vi "Convert Array_String to String.vi"(10 "Data 2":string[][](array[string]), 11 "Data 1":string[](array[string])) -> (3 "String Out":string)   [LabVIEW 2020, in "GUCalibration2.lvlib"]
uses:
  GUCalibration2.lvlib
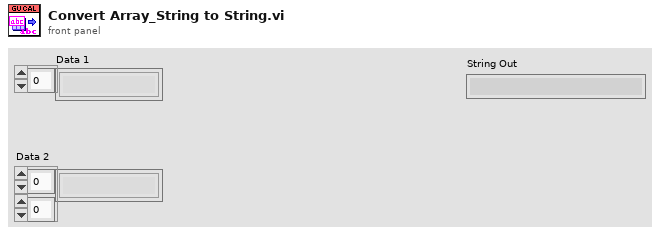
[diagram p1: front panel]
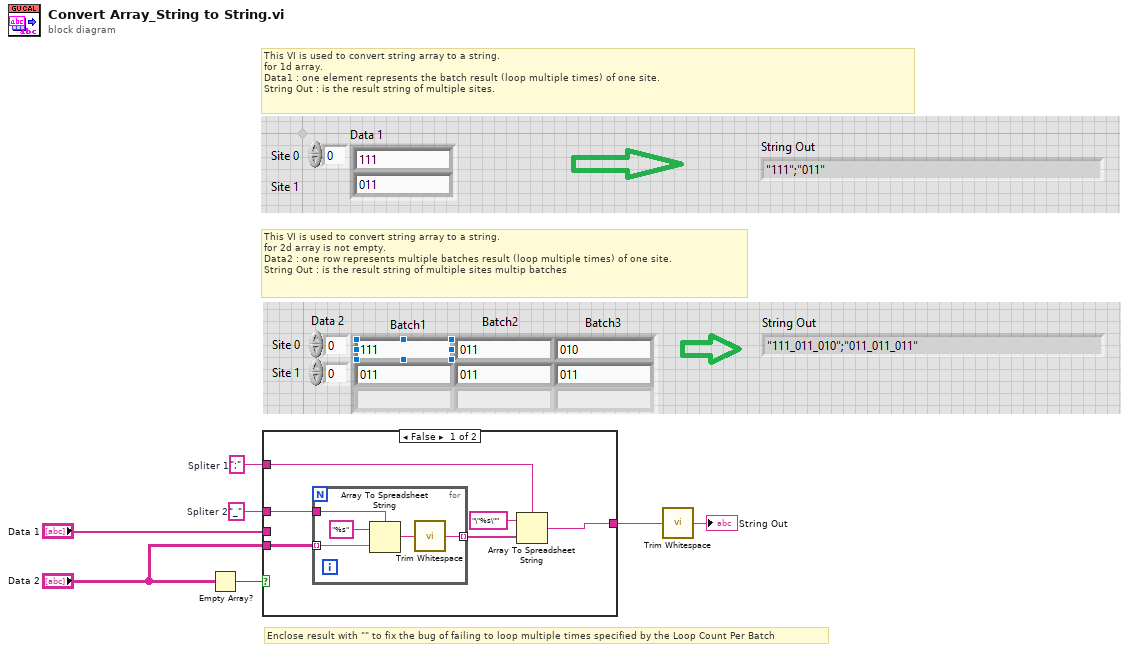
[diagram p0: block diagram]
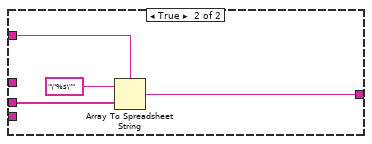
[diagram p2: hidden frame]
diagram:
  w3 = "_"  # Spliter 2
  w4 = ";"  # Spliter 1
  # "This VI is used to convert string array to a string.\nfor 2d array is not empty.\nData2 : one row represents multiple batches result (loop multiple times) of one site.\nString Out : is the result string of multiple sites multip batches"
  # "This VI is used to convert string array to a string.\nfor 1d array.\nData1 : one element represents the batch result (loop multiple times) of one site.\nString Out : is the result string of multiple sites."
  # "Enclose result with \"\" to fix the bug of failing to loop multiple times specified by the Loop Count Per Batch"
  n1 = Empty Array?(array="Data 2") -> (empty?=w5:bool)
  n2 = case shown="False" w5 {
    tunnel: "Data 1" -> [_ w22]
    tunnel: w3 -> [w12 _]
    tunnel: "Data 2" -> [w13 _]
    tunnel: w4 -> [w11 w20]
    tunnel: [w8 w19] -> w2
    frame False {
      n3 = for {
        tunnel: w13 -> [w17] mode=indexing
        tunnel: w12 -> [w16]
        tunnel: [w14] -> w9 mode=indexing
        n4 = Array To Spreadsheet String(delimiter (Tab)=w16, array=w17, 3:"%s" ("format string")) -> (spreadsheet string=w15:string)
        n5 = call <vilib>:"Trim Whitespace.vi"("string"=w15) -> ("trimmed string"=w14:string)  [unwired: 1 in]
      }
      n6 = Array To Spreadsheet String(delimiter (Tab)=w11, array=w9, 3:"\"%s\"" ("format string")) -> (spreadsheet string=w8:string)
    }
    frame True {
      n7 = Array To Spreadsheet String(delimiter (Tab)=w20, array=w22, 3:"\"%s\"" ("format string")) -> (spreadsheet string=w19:string)
    }
  }
  n8 = call <vilib>:"Trim Whitespace.vi"("string"=w2) -> ("trimmed string"=→"String Out":string)  [unwired: 1 in]
